vi "create_NG_folder.vi"(11 "output folder in":path) -> (3 "NG folder array":string[](array[string]))   [LabVIEW 2017]
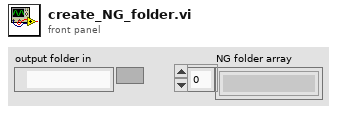
[diagram p1: front panel]
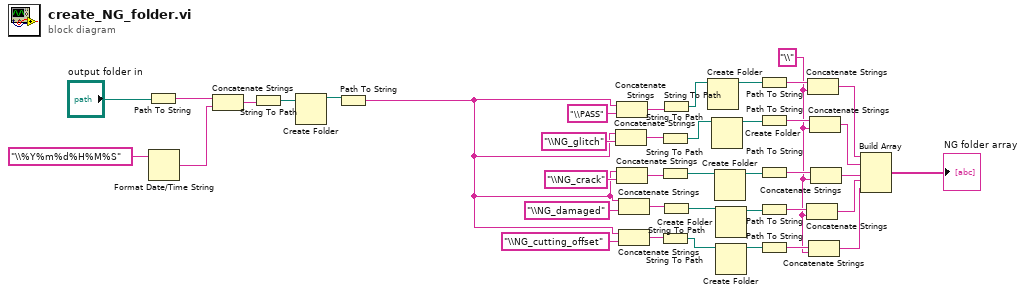
[diagram p0: block diagram]
diagram:
  w12 = "\\" ("string")
  n1 = Path To String(path="output folder in") -> (string=w6:string)
  n2 = Format Date/Time String(time format string (%c)="\\%Y%m%d%H%M%S") -> (date/time string=w5:string)  [unwired: 2 in]
  n3 = Concatenate Strings(w6, w5) -> (w4:string)
  n4 = String To Path(string=w4) -> (path=w3:path)
  n5 = Create Folder(path (use dialog)=w3) -> (created path=w2:path)  [unwired: 2 in, 2 out]
  n6 = Path To String(path=w2) -> (string=w1:string)
  n7 = Concatenate Strings(w1, "\\NG_glitch" ("string")) -> (w32:string)
  n8 = Concatenate Strings(w1, "\\PASS" ("string")) -> (w26:string)
  n9 = Concatenate Strings(w1, "\\NG_crack" ("string")) -> (w34:string)
  n10 = Concatenate Strings(w1, "\\NG_damaged" ("string")) -> (w35:string)
  n11 = Concatenate Strings(w1, "\\NG_cutting_offset" ("string")) -> (w36:string)
  n12 = String To Path(string=w32) -> (path=w33:path)
  n13 = String To Path(string=w34) -> (path=w37:path)
  n14 = String To Path(string=w36) -> (path=w39:path)
  n15 = String To Path(string=w26) -> (path=w25:path)
  n16 = String To Path(string=w35) -> (path=w38:path)
  n17 = Create Folder(path (use dialog)=w25) -> (created path=w23:path)  [unwired: 2 in, 2 out]
  n18 = Create Folder(path (use dialog)=w33) -> (created path=w22:path)  [unwired: 2 in, 2 out]
  n19 = Create Folder(path (use dialog)=w37) -> (created path=w21:path)  [unwired: 2 in, 2 out]
  n20 = Create Folder(path (use dialog)=w38) -> (created path=w20:path)  [unwired: 2 in, 2 out]
  n21 = Create Folder(path (use dialog)=w39) -> (created path=w19:path)  [unwired: 2 in, 2 out]
  n22 = Path To String(path=w23) -> (string=w18:string)
  n23 = Path To String(path=w22) -> (string=w16:string)
  n24 = Path To String(path=w21) -> (string=w15:string)
  n25 = Path To String(path=w20) -> (string=w14:string)
  n26 = Path To String(path=w19) -> (string=w13:string)
  n27 = Concatenate Strings(w14, w12) -> (w9:string)
  n28 = Concatenate Strings(w18, w12) -> (w11:string)
  n29 = Concatenate Strings(w13, w12) -> (w8:string)
  n30 = Concatenate Strings(w16, w12) -> (w10:string)
  n31 = Concatenate Strings(w15, w12) -> (w17:string)
  n32 = Build Array(w11, w10, w17, w9, w8) -> (→"NG folder array":string[])
